vi "SQL获取数据.vi"() -> ()   [LabVIEW 2017]
panel:
  in  "TestMessage Delete":string
  in  "ProssureType Delete":string
  in  "ProductNumber Delete":string
  out "子数组":string[](array[string])
  in  "WorkNumber Delete":string
  out "连接的字符串 2":string
  out "Data":string[][](array[string])
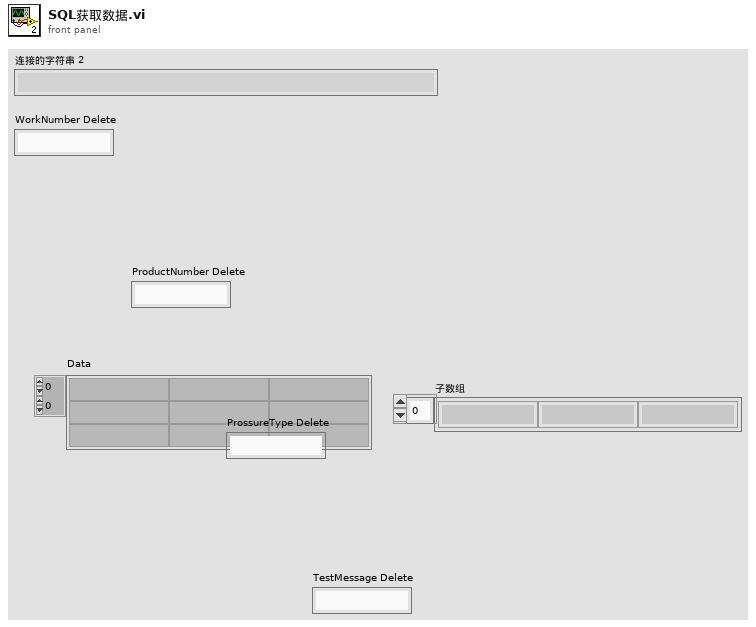
[diagram p1: front panel]
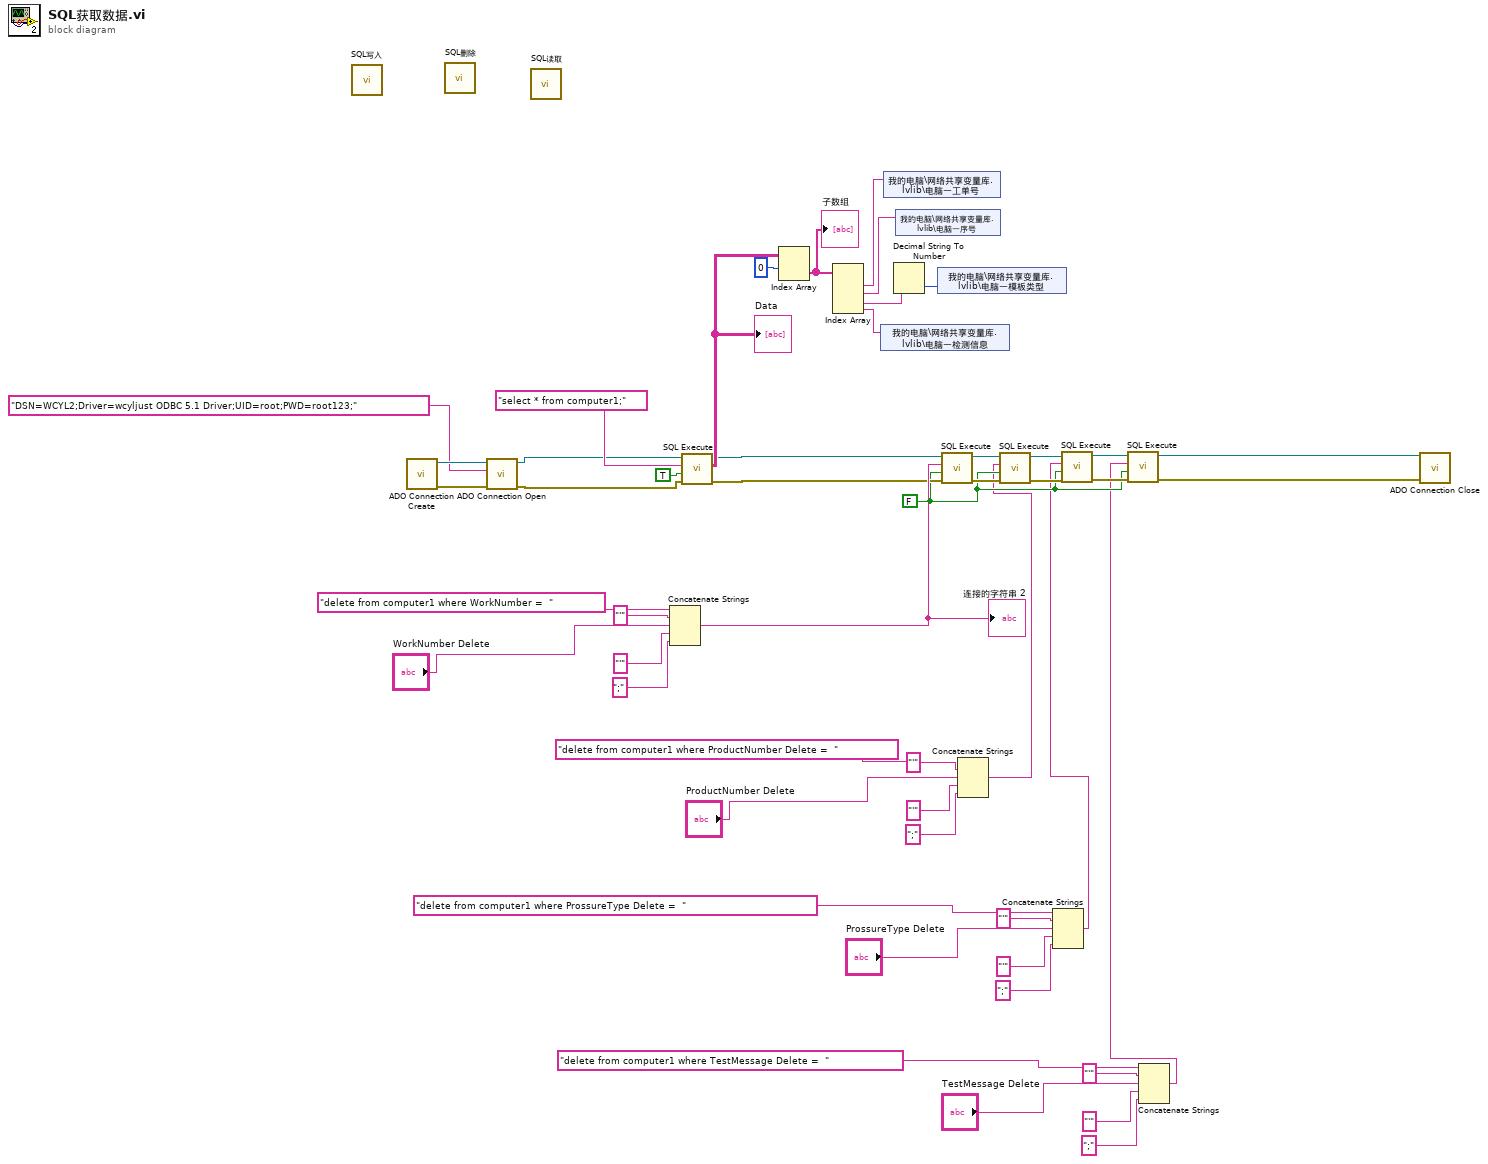
[diagram p0: block diagram]
diagram:
  w9 = FALSE ("Return Data (T)")
  n1 = call "SQL写入.vi"() -> ()  [unwired: 15 in, 1 out]
  n2 = call <userlib>:"ADO Connection Create.vi"() -> ("error out"=w4:errorcluster, "ADODB._Connection Out"=w5:refnum<k7>)  [unwired: 10 in]
  n3 = call "SQL删除.vi"() -> ()  [unwired: 15 in, 1 out]
  n4 = call <userlib>:"ADO Connection Open.vi"("error in (no error)"=w4, "ConnectionString"="DSN=WCYL2;Driver=wcyljust ODBC 5.1 Driver;UID=root;PWD=root123;", "ADODB._Connection In"=w5) -> ("error out"=w1:errorcluster, "ADODB._Connection Out"=w2:refnum<k7>)  [unwired: 7 in]
  n5 = call "SQL读取.vi"() -> ()  [unwired: 10 in, 2 out]
  n6 = Concatenate Strings("delete from computer1 where WorkNumber =  " ("Command Text"), "'" ("字符串"), "WorkNumber Delete", "'" ("字符串"), ";" ("字符串")) -> (w41:string)
  "连接的字符串 2" <- w41
  n7 = call <userlib>:"SQL Execute.vi"("error in (no error)"=w1, "Return Data (T)"=TRUE, "Command Text"="select * from computer1;", "ADODB._Connection In"=w2) -> ("error out"=w37:errorcluster, "Data"=w46:string[][], "ADODB._Connection Out"=w38:refnum<k7>)  [unwired: 4 in, 1 out]
  "Data" <- w46
  n8 = Index Array(array=w46, index (row)=0 ("索引 (行)")) -> (element=w49:string[])  [unwired: 1 in]
  "子数组" <- w49
  n9 = Index Array(array=w49) -> (element #1=w50:string, element #2=w48:string, element #3=w35:string, element #4=w36:string)  [unwired: 4 in]
  n10 = shared-variable "我的电脑\\网络共享变量库.lvlib\\电脑一检测信息"(w36) -> ()  [unwired: 1 in, 1 out]
  n11 = shared-variable "我的电脑\\网络共享变量库.lvlib\\电脑一工单号"(w50) -> ()  [unwired: 1 in, 1 out]
  n12 = Decimal String To Number(string=w35) -> (number=w34:i32)  [unwired: 2 in, 1 out]
  n13 = shared-variable "我的电脑\\网络共享变量库.lvlib\\电脑一序号"(w48) -> ()  [unwired: 1 in, 1 out]
  n14 = shared-variable "我的电脑\\网络共享变量库.lvlib\\电脑一模板类型"(w34) -> ()  [unwired: 1 in, 1 out]
  n15 = call <userlib>:"SQL Execute.vi"("error in (no error)"=w37, "Return Data (T)"=w9, "Command Text"=w41, "ADODB._Connection In"=w38) -> ("error out"=w13:errorcluster, "ADODB._Connection Out"=w17:refnum<k7>)  [unwired: 4 in, 2 out]
  n16 = Concatenate Strings("delete from computer1 where ProductNumber Delete =  " ("Command Text"), "'" ("字符串"), "ProductNumber Delete", "'" ("字符串"), ";" ("字符串")) -> (w8:string)
  n17 = call <userlib>:"SQL Execute.vi"("error in (no error)"=w13, "Return Data (T)"=w9, "Command Text"=w8, "ADODB._Connection In"=w17) -> ("error out"=w12:errorcluster, "ADODB._Connection Out"=w16:refnum<k7>)  [unwired: 4 in, 2 out]
  n18 = Concatenate Strings("delete from computer1 where ProssureType Delete =  " ("Command Text"), "'" ("字符串"), "ProssureType Delete", "'" ("字符串"), ";" ("字符串")) -> (w7:string)
  n19 = call <userlib>:"SQL Execute.vi"("error in (no error)"=w12, "Return Data (T)"=w9, "Command Text"=w7, "ADODB._Connection In"=w16) -> ("error out"=w11:errorcluster, "ADODB._Connection Out"=w15:refnum<k7>)  [unwired: 4 in, 2 out]
  n20 = Concatenate Strings("delete from computer1 where TestMessage Delete =  " ("Command Text"), "'" ("字符串"), "TestMessage Delete", "'" ("字符串"), ";" ("字符串")) -> (w6:string)
  n21 = call <userlib>:"SQL Execute.vi"("error in (no error)"=w11, "Return Data (T)"=w9, "Command Text"=w6, "ADODB._Connection In"=w15) -> ("error out"=w10:errorcluster, "ADODB._Connection Out"=w14:refnum<k7>)  [unwired: 4 in, 2 out]
  n22 = call <userlib>:"ADO Connection Close.vi"("error in (no error)"=w10, "ADODB._Connection In"=w14) -> ()  [unwired: 8 in, 2 out]
